vi "FipsAdjacent.vi"() -> (11 "Fips":i32[](array[numeric]))   [LabVIEW 2017] (continued)
26157\n\"Schoolcraft County, MI\"\t26153\t\"Alger County, MI\"\t26003\n\"Schoolcraft County, MI\"\t26153\t\"Charlevoix County, MI\"\t26029\n\"Schoolcraft County, MI\"\t26153\t\"Delta County, MI\"\t26041\n\"Schoolcraft County, MI\"\t26153\t\"Leelanau County, MI\"\t26089\n\"Schoolcraft County, MI\"\t26153\t\"Luce County, MI\"\t26095\n\"Schoolcraft County, MI\"\t26153\t\"Mackinac County, MI\"\t26097\n\"Schoolcraft County, MI\"\t26153\t\"Schoolcraft County, MI\"\t26153\n\"Shiawassee County, MI\"\t26155\t\"Clinton County, MI\"\t26037\n\"Shiawassee County, MI\"\t26155\t\"Genesee County, MI\"\t26049\n\"Shiawassee County, MI\"\t26155\t\"Gratiot County, MI\"\t26057\n\"Shiawassee County, MI\"\t26155\t\"Ingham County, MI\"\t26065\n\"Shiawassee County, MI\"\t26155\t\"Livingston County, MI\"\t26093\n\"Shiawassee County, MI\"\t26155\t\"Saginaw County, MI\"\t26145\n\"Shiawassee County, MI\"\t26155\t\"Shiawassee County, MI\"\t26155\n\"Tuscola County, MI\"\t26157\t\"Bay County, MI\"\t26017\n\"Tuscola County, MI\"\t26157\t\"Genesee County, MI\"\t26049\n\"Tuscola County, MI\"\t26157\t\"Huron County, MI\"\t26063\n\"Tuscola County, MI\"\t26157\t\"Lapeer County, MI\"\t26087\n\"Tuscola County, MI\"\t26157\t\"Saginaw County, MI\"\t26145\n\"Tuscola County, MI\"\t26157\t\"Sanilac County, MI\"\t26151\n\"Tuscola County, MI\"\t26157\t\"Tuscola County, MI\"\t26157\n\"Van Buren County, MI\"\t26159\t\"Lake County, IL\"\t17097\n\"Van Buren County, MI\"\t26159\t\"Allegan County, MI\"\t26005\n\"Van Buren County, MI\"\t26159\t\"Berrien County, MI\"\t26021\n\"Van Buren County, MI\"\t26159\t\"Cass County, MI\"\t26027\n\"Van Buren County, MI\"\t26159\t\"Kalamazoo County, MI\"\t26077\n\"Van Buren County, MI\"\t26159\t\"St. Joseph County, MI\"\t26149\n\"Van Buren County, MI\"\t26159\t\"Van Buren County, MI\"\t26159\n\"Washtenaw County, MI\"\t26161\t\"Jackson County, MI\"\t26075\n\"Washtenaw County, MI\"\t26161\t\"Lenawee County, MI\"\t26091\n\"Washtenaw County, MI\"\t26161\t\"Livingston County, MI\"\t26093\n\"Washtenaw County, MI\"\t26161\t\"Monroe County, MI\"\t26115\n\"Washtenaw County, MI\"\t26161\t\"Oakland County, MI\"\t26125\n\"Washtenaw County, MI\"\t26161\t\"Washtenaw County, MI\"\t26161\n\"Washtenaw County, MI\"\t26161\t\"Wayne County, MI\"\t26163\n\"Wayne County, MI\"\t26163\t\"Macomb County, MI\"\t26099\n\"Wayne County, MI\"\t26163\t\"Monroe County, MI\"\t26115\n\"Wayne County, MI\"\t26163\t\"Oakland County, MI\"\t26125\n\"Wayne County, MI\"\t26163\t\"Washtenaw County, MI\"\t26161\n\"Wayne County, MI\"\t26163\t\"Wayne County, MI\"\t26163\n\"Wexford County, MI\"\t26165\t\"Benzie County, MI\"\t26019\n\"Wexford County, MI\"\t26165\t\"Grand Traverse County, MI\"\t26055\n\"Wexford County, MI\"\t26165\t\"Kalkaska County, MI\"\t26079\n\"Wexford County, MI\"\t26165\t\"Lake County, MI\"\t26085\n\"Wexford County, MI\"\t26165\t\"Manistee County, MI\"\t26101\n\"Wexford County, MI\"\t26165\t\"Missaukee County, MI\"\t26113\n\"Wexford County, MI\"\t26165\t\"Osceola County, MI\"\t26133\n\"Wexford County, MI\"\t26165\t\"Wexford County, MI\"\t26165\n\"Aitkin County, MN\"\t27001\t\"Aitkin County, MN\"\t27001\n\"Aitkin County, MN\"\t27001\t\"Carlton County, MN\"\t27017\n\"Aitkin County, MN\"\t27001\t\"Cass County, MN\"\t27021\n\"Aitkin County, MN\"\t27001\t\"Crow Wing County, MN\"\t27035\n\"Aitkin County, MN\"\t27001\t\"Itasca County, MN\"\t27061\n\"Aitkin County, MN\"\t27001\t\"Kanabec County, MN\"\t27065\n\"Aitkin County, MN\"\t27001\t\"Mille Lacs County, MN\"\t27095\n\"Aitkin County, MN\"\t27001\t\"Pine County, MN\"\t27115\n\"Aitkin County, MN\"\t27001\t\"St. Louis County, MN\"\t27137\n\"Anoka County, MN\"\t27003\t\"Anoka County, MN\"\t27003\n\"Anoka County, MN\"\t27003\t\"Chisago County, MN\"\t27025\n\"Anoka County, MN\"\t27003\t\"Hennepin County, MN\"\t27053\n\"Anoka County, MN\"\t27003\t\"Isanti County, MN\"\t27059\n\"Anoka County, MN\"\t27003\t\"Ramsey County, MN\"\t27123\n\"Anoka County, MN\"\t27003\t\"Sherburne County, MN\"\t27141\n\"Anoka County, MN\"\t27003\t\"Washington County, MN\"\t27163\n\"Becker County, MN\"\t27005\t\"Becker County, MN\"\t27005\n\"Becker County, MN\"\t27005\t\"Clay County, MN\"\t27027\n\"Becker County, MN\"\t27005\t\"Clearwater County, MN\"\t27029\n\"Becker County, MN\"\t27005\t\"Hubbard County, MN\"\t27057\n\"Becker County, MN\"\t27005\t\"Mahnomen County, MN\"\t27087\n\"Becker County, MN\"\t27005\t\"Norman County, MN\"\t27107\n\"Becker County, MN\"\t27005\t\"Otter Tail County, MN\"\t27111\n\"Becker County, MN\"\t27005\t\"Wadena County, MN\"\t27159\n\"Beltrami County, MN\"\t27007\t\"Beltrami County, MN\"\t27007\n\"Beltrami County, MN\"\t27007\t\"Cass County, MN\"\t27021\n\"Beltrami County, MN\"\t27007\t\"Clearwater County, MN\"\t27029\n\"Beltrami County, MN\"\t27007\t\"Hubbard County, MN\"\t27057\n\"Beltrami County, MN\"\t27007\t\"Itasca County, MN\"\t27061\n\"Beltrami County, MN\"\t27007\t\"Koochiching County, MN\"\t27071\n\"Beltrami County, MN\"\t27007\t\"Lake of the Woods County, MN\"\t27077\n\"Beltrami County, MN\"\t27007\t\"Marshall County, MN\"\t27089\n\"Beltrami County, MN\"\t27007\t\"Pennington County, MN\"\t27113\n\"Beltrami County, MN\"\t27007\t\"Roseau County, MN\"\t27135\n\"Benton County, MN\"\t27009\t\"Benton County, MN\"\t27009\n\"Benton County, MN\"\t27009\t\"Mille Lacs County, MN\"\t27095\n\"Benton County, MN\"\t27009\t\"Morrison County, MN\"\t27097\n\"Benton County, MN\"\t27009\t\"Sherburne County, MN\"\t27141\n\"Benton County, MN\"\t27009\t\"Stearns County, MN\"\t27145\n\"Big Stone County, MN\"\t27011\t\"Big Stone County, MN\"\t27011\n\"Big Stone County, MN\"\t27011\t\"Lac qui Parle County, MN\"\t27073\n\"Big Stone County, MN\"\t27011\t\"Stevens County, MN\"\t27149\n\"Big Stone County, MN\"\t27011\t\"Swift County, MN\"\t27151\n\"Big Stone County, MN\"\t27011\t\"Traverse County, MN\"\t27155\n\"Big Stone County, MN\"\t27011\t\"Grant County, SD\"\t46051\n\"Big Stone County, MN\"\t27011\t\"Roberts County, SD\"\t46109\n\"Blue Earth County, MN\"\t27013\t\"Blue Earth County, MN\"\t27013\n\"Blue Earth County, MN\"\t27013\t\"Brown County, MN\"\t27015\n\"Blue Earth County, MN\"\t27013\t\"Faribault County, MN\"\t27043\n\"Blue Earth County, MN\"\t27013\t\"Le Sueur County, MN\"\t27079\n\"Blue Earth County, MN\"\t27013\t\"Martin County, MN\"\t27091\n\"Blue Earth County, MN\"\t27013\t\"Nicollet County, MN\"\t27103\n\"Blue Earth County, MN\"\t27013\t\"Waseca County, MN\"\t27161\n\"Blue Earth County, MN\"\t27013\t\"Watonwan County, MN\"\t27165\n\"Brown County, MN\"\t27015\t\"Blue Earth County, MN\"\t27013\n\"Brown County, MN\"\t27015\t\"Brown County, MN\"\t27015\n\"Brown County, MN\"\t27015\t\"Cottonwood County, MN\"\t27033\n\"Brown County, MN\"\t27015\t\"Nicollet County, MN\"\t27103\n\"Brown County, MN\"\t27015\t\"Redwood County, MN\"\t27127\n\"Brown County, MN\"\t27015\t\"Renville County, MN\"\t27129\n\"Brown County, MN\"\t27015\t\"Watonwan County, MN\"\t27165\n\"Carlton County, MN\"\t27017\t\"Aitkin County, MN\"\t27001\n\"Carlton County, MN\"\t27017\t\"Carlton County, MN\"\t27017\n\"Carlton County, MN\"\t27017\t\"Pine County, MN\"\t27115\n\"Carlton County, MN\"\t27017\t\"St. Louis County, MN\"\t27137\n\"Carlton County, MN\"\t27017\t\"Douglas County, WI\"\t55031\n\"Carver County, MN\"\t27019\t\"Carver County, MN\"\t27019\n\"Carver County, MN\"\t27019\t\"Hennepin County, MN\"\t27053\n\"Carver County, MN\"\t27019\t\"McLeod County, MN\"\t27085\n\"Carver County, MN\"\t27019\t\"Scott County, MN\"\t27139\n\"Carver County, MN\"\t27019\t\"Sibley County, MN\"\t27143\n\"Carver County, MN\"\t27019\t\"Wright County, MN\"\t27171\n\"Cass County, MN\"\t27021\t\"Aitkin County, MN\"\t27001\n\"Cass County, MN\"\t27021\t\"Beltrami County, MN\"\t27007\n\"Cass County, MN\"\t27021\t\"Cass County, MN\"\t27021\n\"Cass County, MN\"\t27021\t\"Crow Wing County, MN\"\t27035\n\"Cass County, MN\"\t27021\t\"Hubbard County, MN\"\t27057\n\"Cass County, MN\"\t27021\t\"Itasca County, MN\"\t27061\n\"Cass County, MN\"\t27021\t\"Morrison County, MN\"\t27097\n\"Cass County, MN\"\t27021\t\"Todd County, MN\"\t27153\n\"Cass County, MN\"\t27021\t\"Wadena County, MN\"\t27159\n\"Chippewa County, MN\"\t27023\t\"Chippewa County, MN\"\t27023\n\"Chippewa County, MN\"\t27023\t\"Kandiyohi County, MN\"\t27067\n\"Chippewa County, MN\"\t27023\t\"Lac qui Parle County, MN\"\t27073\n\"Chippewa County, MN\"\t27023\t\"Renville County, MN\"\t27129\n\"Chippewa County, MN\"\t27023\t\"Swift County, MN\"\t27151\n\"Chippewa County, MN\"\t27023\t\"Yellow Medicine County, MN\"\t27173\n\"Chisago County, MN\"\t27025\t\"Anoka County, MN\"\t27003\n\"Chisago County, MN\"\t27025\t\"Chisago County, MN\"\t27025\n\"Chisago County, MN\"\t27025\t\"Isanti County, MN\"\t27059\n\"Chisago County, MN\"\t27025\t\"Kanabec County, MN\"\t27065\n\"Chisago County, MN\"\t27025\t\"Pine County, MN\"\t27115\n\"Chisago County, MN\"\t27025\t\"Washington County, MN\"\t27163\n\"Chisago County, MN\"\t27025\t\"Burnett County, WI\"\t55013\n\"Chisago County, MN\"\t27025\t\"Polk County, WI\"\t55095\n\"Clay County, MN\"\t27027\t\"Becker County, MN\"\t27005\n\"Clay County, MN\"\t27027\t\"Clay County, MN\"\t27027\n\"Clay County, MN\"\t27027\t\"Norman County, MN\"\t27107\n\"Clay County, MN\"\t27027\t\"Otter Tail County, MN\"\t27111\n\"Clay County, MN\"\t27027\t\"Wilkin County, MN\"\t27167\n\"Clay County, MN\"\t27027\t\"Cass County, ND\"\t38017\n\"Clay County, MN\"\t27027\t\"Richland County, ND\"\t38077\n\"Clearwater County, MN\"\t27029\t\"Becker County, MN\"\t27005\n\"Clearwater County, MN\"\t27029\t\"Beltrami County, MN\"\t27007\n\"Clearwater County, MN\"\t27029\t\"Clearwater County, MN\"\t27029\n\"Clearwater County, MN\"\t27029\t\"Hubbard County, MN\"\t27057\n\"Clearwater County, MN\"\t27029\t\"Mahnomen County, MN\"\t27087\n\"Clearwater County, MN\"\t27029\t\"Pennington County, MN\"\t27113\n\"Clearwater County, MN\"\t27029\t\"Polk County, MN\"\t27119\n\"Cook County, MN\"\t27031\t\"Keweenaw County, MI\"\t26083\n\"Cook County, MN\"\t27031\t\"Ontonagon County, MI\"\t26131\n\"Cook County, MN\"\t27031\t\"Cook County, MN\"\t27031\n\"Cook County, MN\"\t27031\t\"Lake County, MN\"\t27075\n\"Cook County, MN\"\t27031\t\"Ashland County, WI\"\t55003\n\"Cottonwood County, MN\"\t27033\t\"Brown County, MN\"\t27015\n\"Cottonwood County, MN\"\t27033\t\"Cottonwood County, MN\"\t27033\n\"Cottonwood County, MN\"\t27033\t\"Jackson County, MN\"\t27063\n\"Cottonwood County, MN\"\t27033\t\"Murray County, MN\"\t27101\n\"Cottonwood County, MN\"\t27033\t\"Nobles County, MN\"\t27105\n\"Cottonwood County, MN\"\t27033\t\"Redwood County, MN\"\t27127\n\"Cottonwood County, MN\"\t27033\t\"Watonwan County, MN\"\t27165\n\"Crow Wing County, MN\"\t27035\t\"Aitkin County, MN\"\t27001\n\"Crow Wing County, MN\"\t27035\t\"Cass County, MN\"\t27021\n\"Crow Wing County, MN\"\t27035\t\"Crow Wing County, MN\"\t27035\n\"Crow Wing County, MN\"\t27035\t\"Mille Lacs County, MN\"\t27095\n\"Crow Wing County, MN\"\t27035\t\"Morrison County, MN\"\t27097\n\"Dakota County, MN\"\t27037\t\"Dakota County, MN\"\t27037\n\"Dakota County, MN\"\t27037\t\"Goodhue County, MN\"\t27049\n\"Dakota County, MN\"\t27037\t\"Hennepin County, MN\"\t27053\n\"Dakota County, MN\"\t27037\t\"Ramsey County, MN\"\t27123\n\"Dakota County, MN\"\t27037\t\"Rice County, MN\"\t27131\n\"Dakota County, MN\"\t27037\t\"Scott County, MN\"\t27139\n\"Dakota County, MN\"\t27037\t\"Washington County, MN\"\t27163\n\"Dakota County, MN\"\t27037\t\"Pierce County, WI\"\t55093\n\"Dodge County, MN\"\t27039\t\"Dodge County, MN\"\t27039\n\"Dodge County, MN\"\t27039\t\"Goodhue County, MN\"\t27049\n\"Dodge County, MN\"\t27039\t\"Mower County, MN\"\t27099\n\"Dodge County, MN\"\t27039\t\"Olmsted County, MN\"\t27109\n\"Dodge County, MN\"\t27039\t\"Rice County, MN\"\t27131\n\"Dodge County, MN\"\t27039\t\"Steele County, MN\"\t27147\n\"Douglas County, MN\"\t27041\t\"Douglas County, MN\"\t27041\n\"Douglas County, MN\"\t27041\t\"Grant County, MN\"\t27051\n\"Douglas County, MN\"\t27041\t\"Otter Tail County, MN\"\t27111\n\"Douglas County, MN\"\t27041\t\"Pope County, MN\"\t27121\n\"Douglas County, MN\"\t27041\t\"Stearns County, MN\"\t27145\n\"Douglas County, MN\"\t27041\t\"Stevens County, MN\"\t27149\n\"Douglas County, MN\"\t27041\t\"Todd County, MN\"\t27153\n\"Faribault County, MN\"\t27043\t\"Kossuth County, IA\"\t19109\n\"Faribault County, MN\"\t27043\t\"Winnebago County, IA\"\t19189\n\"Faribault County, MN\"\t27043\t\"Blue Earth County, MN\"\t27013\n\"Faribault County, MN\"\t27043\t\"Faribault County, MN\"\t27043\n\"Faribault County, MN\"\t27043\t\"Freeborn County, MN\"\t27047\n\"Faribault County, MN\"\t27043\t\"Martin County, MN\"\t27091\n\"Faribault County, MN\"\t27043\t\"Waseca County, MN\"\t27161\n\"Fillmore County, MN\"\t27045\t\"Howard County, IA\"\t19089\n\"Fillmore County, MN\"\t27045\t\"Winneshiek County, IA\"\t19191\n\"Fillmore County, MN\"\t27045\t\"Fillmore County, MN\"\t27045\n\"Fillmore County, MN\"\t27045\t\"Houston County, MN\"\t27055\n\"Fillmore County, MN\"\t27045\t\"Mower County, MN\"\t27099\n\"Fillmore County, MN\"\t27045\t\"Olmsted County, MN\"\t27109\n\"Fillmore County, MN\"\t27045\t\"Winona County, MN\"\t27169\n\"Freeborn County, MN\"\t27047\t\"Winnebago County, IA\"\t19189\n\"Freeborn County, MN\"\t27047\t\"Worth County, IA\"\t19195\n\"Freeborn County, MN\"\t27047\t\"Faribault County, MN\"\t27043\n\"Freeborn County, MN\"\t27047\t\"Freeborn County, MN\"\t27047\n\"Freeborn County, MN\"\t27047\t\"Mower County, MN\"\t27099\n\"Freeborn County, MN\"\t27047\t\"Steele County, MN\"\t27147\n\"Freeborn County, MN\"\t27047\t\"Waseca County, MN\"\t27161\n\"Goodhue County, MN\"\t27049\t\"Dakota County, MN\"\t27037\n\"Goodhue County, MN\"\t27049\t\"Dodge County, MN\"\t27039\n\"Goodhue County, MN\"\t27049\t\"Goodhue County, MN\"\t27049\n\"Goodhue County, MN\"\t27049\t\"Olmsted County, MN\"\t27109\n\"Goodhue County, MN\"\t27049\t\"Rice County, MN\"\t27131\n\"Goodhue County, MN\"\t27049\t\"Wabasha County, MN\"\t27157\n\"Goodhue County, MN\"\t27049\t\"Pepin County, WI\"\t55091\n\"Goodhue County, MN\"\t27049\t\"Pierce County, WI\"\t55093\n\"Grant County, MN\"\t27051\t\"Douglas County, MN\"\t27041\n\"Grant County, MN\"\t27051\t\"Grant County, MN\"\t27051\n\"Grant County, MN\"\t27051\t\"Otter Tail County, MN\"\t27111\n\"Grant County, MN\"\t27051\t\"Pope County, MN\"\t27121\n\"Grant County, MN\"\t27051\t\"Stevens County, MN\"\t27149\n\"Grant County, MN\"\t27051\t\"Traverse County, MN\"\t27155\n\"Grant County, MN\"\t27051\t\"Wilkin County, MN\"\t27167\n\"Hennepin County, MN\"\t27053\t\"Anoka County, MN\"\t27003\n\"Hennepin County, MN\"\t27053\t\"Carver County, MN\"\t27019\n\"Hennepin County, MN\"\t27053\t\"Dakota County, MN\"\t27037\n\"Hennepin County, MN\"\t27053\t\"Hennepin County, MN\"\t27053\n\"Hennepin County, MN\"\t27053\t\"Ramsey County, MN\"\t27123\n\"Hennepin County, MN\"\t27053\t\"Scott County, MN\"\t27139\n\"Hennepin County, MN\"\t27053\t\"Sherburne County, MN\"\t27141\n\"Hennepin County, MN\"\t27053\t\"Wright County, MN\"\t27171\n\"Houston County, MN\"\t27055\t\"Allamakee County, IA\"\t19005\n\"Houston County, MN\"\t27055\t\"Winneshiek County, IA\"\t19191\n\"Houston County, MN\"\t27055\t\"Fillmore County, MN\"\t27045\n\"Houston County, MN\"\t27055\t\"Houston County, MN\"\t27055\n\"Houston County, MN\"\t27055\t\"Winona County, MN\"\t27169\n\"Houston County, MN\"\t27055\t\"La Crosse County, WI\"\t55063\n\"Houston County, MN\"\t27055\t\"Vernon County, WI\"\t55123\n\"Hubbard County, MN\"\t27057\t\"Becker County, MN\"\t27005\n\"Hubbard County, MN\"\t27057\t\"Beltrami County, MN\"\t27007\n\"Hubbard County, MN\"\t27057\t\"Cass County, MN\"\t27021\n\"Hubbard County, MN\"\t27057\t\"Clearwater County, MN\"\t27029\n\"Hubbard County, MN\"\t27057\t\"Hubbard County, MN\"\t27057\n\"Hubbard County, MN\"\t27057\t\"Wadena County, MN\"\t27159\n\"Isanti County, MN\"\t27059\t\"Anoka County, MN\"\t27003\n\"Isanti County, MN\"\t27059\t\"Chisago County, MN\"\t27025\n\"Isanti County, MN\"\t27059\t\"Isanti County, MN\"\t27059\n\"Isanti County, MN\"\t27059\t\"Kanabec County, MN\"\t27065\n\"Isanti County, MN\"\t27059\t\"Mille Lacs County, MN\"\t27095\n\"Isanti County, MN\"\t27059\t\"Pine County, MN\"\t27115\n\"Isanti County, MN\"\t27059\t\"Sherburne County, MN\"\t27141\n\"Itasca County, MN\"\t27061\t\"Aitkin County, MN\"\t27001\n\"Itasca County, MN\"\t27061\t\"Beltrami County, MN\"\t27007\n\"Itasca County, MN\"\t27061\t\"Cass County, MN\"\t27021\n\"Itasca County, MN\"\t27061\t\"Itasca County, MN\"\t27061\n\"Itasca County, MN\"\t27061\t\"Koochiching County, MN\"\t27071\n\"Itasca County, MN\"\t27061\t\"St. Louis County, MN\"\t27137\n\"Jackson County, MN\"\t27063\t\"Dickinson County, IA\"\t19059\n\"Jackson County, MN\"\t27063\t\"Emmet County, IA\"\t19063\n\"Jackson County, MN\"\t27063\t\"Osceola County, IA\"\t19143\n\"Jackson County, MN\"\t27063\t\"Cottonwood County, MN\"\t27033\n\"Jackson County, MN\"\t27063\t\"Jackson County, MN\"\t27063\n\"Jackson County, MN\"\t27063\t\"Martin County, MN\"\t27091\n\"Jackson County, MN\"\t27063\t\"Nobles County, MN\"\t27105\n\"Jackson County, MN\"\t27063\t\"Watonwan County, MN\"\t27165\n\"Kanabec County, MN\"\t27065\t\"Aitkin County, MN\"\t27001\n\"Kanabec County, MN\"\t27065\t\"Chisago County, MN\"\t27025\n\"Kanabec County, MN\"\t27065\t\"Isanti County, MN\"\t27059\n\"Kanabec County, MN\"\t27065\t\"Kanabec County, MN\"\t27065\n\"Kanabec County, MN\"\t27065\t\"Mille Lacs County, MN\"\t27095\n\"Kanabec County, MN\"\t27065\t\"Pine County, MN\"\t27115\n\"Kandiyohi County, MN\"\t27067\t\"Chippewa County, MN\"\t27023\n\"Kandiyohi County, MN\"\t27067\t\"Kandiyohi County, MN\"\t27067\n\"Kandiyohi County, MN\"\t27067\t\"Meeker County, MN\"\t27093\n\"Kandiyohi County, MN\"\t27067\t\"Pope County, MN\"\t27121\n\"Kandiyohi County, MN\"\t27067\t\"Renville County, MN\"\t27129\n\"Kandiyohi County, MN\"\t27067\t\"Stearns County, MN\"\t27145\n\"Kandiyohi County, MN\"\t27067\t\"Swift County, MN\"\t27151\n\"Kittson County, MN\"\t27069\t\"Kittson County, MN\"\t27069\n\"Kittson County, MN\"\t27069\t\"Marshall County, MN\"\t27089\n\"Kittson County, MN\"\t27069\t\"Roseau County, MN\"\t27135\n\"Kittson County, MN\"\t27069\t\"Pembina County, ND\"\t38067\n\"Koochiching County, MN\"\t27071\t\"Beltrami County, MN\"\t27007\n\"Koochiching County, MN\"\t27071\t\"Itasca County, MN\"\t27061\n\"Koochiching County, MN\"\t27071\t\"Koochiching County, MN\"\t27071\n\"Koochiching County, MN\"\t27071\t\"Lake of the Woods County, MN\"\t27077\n\"Koochiching County, MN\"\t27071\t\"St. Louis County, MN\"\t27137\n\"Lac qui Parle County, MN\"\t27073\t\"Big Stone County, MN\"\t27011\n\"Lac qui Parle County, MN\"\t27073\t\"Chippewa County, MN\"\t27023\n\"Lac qui Parle County, MN\"\t27073\t\"Lac qui Parle County, MN\"\t27073\n\"Lac qui Parle County, MN\"\t27073\t\"Swift County, MN\"\t27151\n\"Lac qui Parle County, MN\"\t27073\t\"Yellow Medicine County, MN\"\t27173\n\"Lac qui Parle County, MN\"\t27073\t\"Deuel County, SD\"\t46039\n\"Lac qui Parle County, MN\"\t27073\t\"Grant County, SD\"\t46051\n\"Lake County, MN\"\t27075\t\"Cook County, MN\"\t27031\n\"Lake County, MN\"\t27075\t\"Lake County, MN\"\t27075\n\"Lake County, MN\"\t27075\t\"St. Louis County, MN\"\t27137\n\"Lake County, MN\"\t27075\t\"Ashland County, WI\"\t55003\n\"Lake County, MN\"\t27075\t\"Bayfield County, WI\"\t55007\n\"Lake County, MN\"\t27075\t\"Douglas County, WI\"\t55031\n\"Lake of the Woods County, MN\"\t27077\t\"Beltrami County, MN\"\t27007\n\"Lake of the Woods County, MN\"\t27077\t\"Koochiching County, MN\"\t27071\n\"Lake of the Woods County, MN\"\t27077\t\"Lake of the Woods County, MN\"\t27077\n\"Lake of the Woods County, MN\"\t27077\t\"Roseau County, MN\"\t27135\n\"Le Sueur County, MN\"\t27079\t\"Blue Earth County, MN\"\t27013\n\"Le Sueur County, MN\"\t27079\t\"Le Sueur County, MN\"\t27079\n\"Le Sueur County, MN\"\t27079\t\"Nicollet County, MN\"\t27103\n\"Le Sueur County, MN\"\t27079\t\"Rice County, MN\"\t27131\n\"Le Sueur County, MN\"\t27079\t\"Scott County, MN\"\t27139\n\"Le Sueur County, MN\"\t27079\t\"Sibley County, MN\"\t27143\n\"Le Sueur County, MN\"\t27079\t\"Waseca County, MN\"\t27161\n\"Lincoln County, MN\"\t27081\t\"Lincoln County, MN\"\t27081\n\"Lincoln County, MN\"\t27081\t\"Lyon County, MN\"\t27083\n\"Lincoln County, MN\"\t27081\t\"Pipestone County, MN\"\t27117\n\"Lincoln County, MN\"\t27081\t\"Yellow Medicine County, MN\"\t27173\n\"Lincoln County, MN\"\t27081\t\"Brookings County, SD\"\t46011\n\"Lincoln County, MN\"\t27081\t\"Deuel County, SD\"\t46039\n\"Lincoln County, MN\"\t27081\t\"Moody County, SD\"\t46101\n\"Lyon County, MN\"\t27083\t\"Lincoln County, MN\"\t27081\n\"Lyon County, MN\"\t27083\t\"Lyon County, MN\"\t27083\n\"Lyon County, MN\"\t27083\t\"Murray County, MN\"\t27101\n\"Lyon County, MN\"\t27083\t\"Pipestone County, MN\"\t27117\n\"Lyon County, MN\"\t27083\t\"Redwood County, MN\"\t27127\n\"Lyon County, MN\"\t27083\t\"Yellow Medicine County, MN\"\t27173\n\"McLeod County, MN\"\t27085\t\"Carver County, MN\"\t27019\n\"McLeod County, MN\"\t27085\t\"McLeod County, MN\"\t27085\n\"McLeod County, MN\"\t27085\t\"Meeker County, MN\"\t27093\n\"McLeod County, MN\"\t27085\t\"Renville County, MN\"\t27129\n\"McLeod County, MN\"\t27085\t\"Sibley County, MN\"\t27143\n\"McLeod County, MN\"\t27085\t\"Wright County, MN\"\t27171\n\"Mahnomen County, MN\"\t27087\t\"Becker County, MN\"\t27005\n\"Mahnomen County, MN\"\t27087\t\"Clearwater County, MN\"\t27029\n\"Mahnomen County, MN\"\t27087\t\"Mahnomen County, MN\"\t27087\n\"Mahnomen County, MN\"\t27087\t\"Norman County, MN\"\t27107\n\"Mahnomen County, MN\"\t27087\t\"Polk County, MN\"\t27119\n\"Marshall County, MN\"\t27089\t\"Beltrami County, MN\"\t27007\n\"Marshall County, MN\"\t27089\t\"Kittson County, MN\"\t27069\n\"Marshall County, MN\"\t27089\t\"Marshall County, MN\"\t27089\n\"Marshall County, MN\"\t27089\t\"Pennington County, MN\"\t27113\n\"Marshall County, MN\"\t27089\t\"Polk County, MN\"\t27119\n\"Marshall County, MN\"\t27089\t\"Roseau County, MN\"\t27135\n\"Marshall County, MN\"\t27089\t\"Grand Forks County, ND\"\t38035\n\"Marshall County, MN\"\t27089\t\"Pembina County, ND\"\t38067\n\"Marshall County, MN\"\t27089\t\"Walsh County, ND\"\t38099\n\"Martin County, MN\"\t27091\t\"Emmet County, IA\"\t19063\n\"Martin County, MN\"\t27091\t\"Kossuth County, IA\"\t19109\n\"Martin County, MN\"\t27091\t\"Blue Earth County, MN\"\t27013\n\"Martin County, MN\"\t27091\t\"Faribault County, MN\"\t27043\n\"Martin County, MN\"\t27091\t\"Jackson County, MN\"\t27063\n\"Martin County, MN\"\t27091\t\"Martin County, MN\"\t27091\n\"Martin County, MN\"\t27091\t\"Watonwan County, MN\"\t27165\n\"Meeker County, MN\"\t27093\t\"Kandiyohi County, MN\"\t27067\n\"Meeker County, MN\"\t27093\t\"McLeod County, MN\"\t27085\n\"Meeker County, MN\"\t27093\t\"Meeker County, MN\"\t27093\n\"Meeker County, MN\"\t27093\t\"Renville County, MN\"\t27129\n\"Meeker County, MN\"\t27093\t\"Stearns County, MN\"\t27145\n\"Meeker County, MN\"\t27093\t\"Wright County, MN\"\t27171\n\"Mille Lacs County, MN\"\t27095\t\"Aitkin County, MN\"\t27001\n\"Mille Lacs County, MN\"\t27095\t\"Benton County, MN\"\t27009\n\"Mille Lacs County, MN\"\t27095\t\"Crow Wing County, MN\"\t27035\n\"Mille Lacs County, MN\"\t27095\t\"Isanti County, MN\"\t27059\n\"Mille Lacs County, MN\"\t27095\t\"Kanabec County, MN\"\t27065\n\"Mille Lacs County, MN\"\t27095\t\"Mille Lacs County, MN\"\t27095\n\"Mille Lacs County, MN\"\t27095\t\"Morrison County, MN\"\t27097\n\"Mille Lacs County, MN\"\t27095\t\"Sherburne County, MN\"\t27141\n\"Morrison County, MN\"\t27097\t\"Benton County, MN\"\t27009\n\"Morrison County, MN\"\t27097\t\"Cass County, MN\"\t27021\n\"Morrison County, MN\"\t27097\t\"Crow Wing County, MN\"\t27035\n\"Morrison County, MN\"\t27097\t\"Mille Lacs County, MN\"\t27095\n\"Morrison County, MN\"\t27097\t\"Morrison County, MN\"\t27097\n\"Morrison County, MN\"\t27097\t\"Stearns County, MN\"\t27145\n\"Morrison County, MN\"\t27097\t\"Todd County, MN\"\t27153\n\"Mower County, MN\"\t27099\t\"Howard County, IA\"\t19089\n\"Mower County, MN\"\t27099\t\"Mitchell County, IA\"\t19131\n\"Mower County, MN\"\t27099\t\"Worth County, IA\"\t19195\n\"Mower County, MN\"\t27099\t\"Dodge County, MN\"\t27039\n\"Mower County, MN\"\t27099\t\"Fillmore County, MN\"\t27045\n\"Mower County, MN\"\t27099\t\"Freeborn County, MN\"\t27047\n\"Mower County, MN\"\t27099\t\"Mower County, MN\"\t27099\n\"Mower County, MN\"\t27099\t\"Olmsted County, MN\"\t27109\n\"Mower County, MN\"\t27099\t\"Steele County, MN\"\t27147\n\"Murray County, MN\"\t27101\t\"Cottonwood County, MN\"\t27033\n\"Murray County, MN\"\t27101\t\"Lyon County, MN\"\t27083\n\"Murray County, MN\"\t27101\t\"Murray County, MN\"\t27101\n\"Murray County, MN\"\t27101\t\"Nobles County, MN\"\t27105\n\"Murray County, MN\"\t27101\t\"Pipestone County, MN\"\t27117\n\"Murray County, MN\"\t27101\t\"Redwood County, MN\"\t27127\n\"Murray County, MN\"\t27101\t\"Rock County, MN\"\t27133\n\"Nicollet County, MN\"\t27103\t\"Blue Earth County, MN\"\t27013\n\"Nicollet County, MN\"\t27103\t\"Brown County, MN\"\t27015\n\"Nicollet County, MN\"\t27103\t\"Le Sueur County, MN\"\t27079\n\"Nicollet County, MN\"\t27103\t\"Nicollet County, MN\"\t27103\n\"Nicollet County, MN\"\t27103\t\"Renville County, MN\"\t27129\n\"Nicollet County, MN\"\t27103\t\"Sibley County, MN\"\t27143\n\"Nobles County, MN\"\t27105\t\"Lyon County, IA\"\t19119\n\"Nobles County, MN\"\t27105\t\"Osceola County, IA\"\t19143\n\"Nobles County, MN\"\t27105\t\"Cottonwood County, MN\"\t27033\n\"Nobles County, MN\"\t27105\t\"Jackson County, MN\"\t27063\n\"Nobles County, MN\"\t27105\t\"Murray County, MN\"\t27101\n\"Nobles County, MN\"\t27105\t\"Nobles County, MN\"\t27105\n\"Nobles County, MN\"\t27105\t\"Rock County, MN\"\t27133\n\"Norman County, MN\"\t27107\t\"Becker County, MN\"\t27005\n\"Norman County, MN\"\t27107\t\"Clay County, MN\"\t27027\n\"Norman County, MN\"\t27107\t\"Mahnomen County, MN\"\t27087\n\"Norman County, MN\"\t27107\t\"Norman County, MN\"\t27107\n\"Norman County, MN\"\t27107\t\"Polk County, MN\"\t27119\n\"Norman County, MN\"\t27107\t\"Cass County, ND\"\t38017\n\"Norman County, MN\"\t27107\t\"Traill County, ND\"\t38097\n\"Olmsted County, MN\"\t27109\t\"Dodge County, MN\"\t27039\n\"Olmsted County, MN\"\t27109\t\"Fillmore County, MN\"\t27045\n\"Olmsted County, MN\"\t27109\t\"Goodhue County, MN\"\t27049\n\"Olmsted County, MN\"\t27109\t\"Mower County, MN\"\t27099\n\"Olmsted County, MN\"\t27109\t\"Olmsted County, MN\"\t27109\n\"Olmsted County, MN\"\t27109\t\"Wabasha County, MN\"\t27157\n\"Olmsted County, MN\"\t27109\t\"Winona County, MN\"\t27169\n\"Todd County, MN\"\t27111\t\"Becker County, MN\"\t27005\n\"Todd County, MN\"\t27111\t\"Clay County, MN\"\t27027\n\"Todd County, MN\"\t27111\t\"Douglas County, MN\"\t27041\n\"Todd County, MN\"\t27111\t\"Grant County, MN\"\t27051\n\"Todd County, MN\"\t27111\t\"Otter Tail County, MN\"\t27111\n\"Todd County, MN\"\t27111\t\"Todd County, MN\"\t27153\n\"Todd County, MN\"\t27111\t\"Wadena County, MN\"\t27159\n\"Todd County, MN\"\t27111\t\"Wilkin County, MN\"\t27167\n\"Pennington County, MN\"\t27113\t\"Beltrami County, MN\"\t27007\n\"Pennington County, MN\"\t27113\t\"Clearwater County, MN\"\t27029\n\"Pennington County, MN\"\t27113\t\"Marshall County, MN\"\t27089\n\"Pennington County, MN\"\t27113\t\"Pennington County, MN\"\t27113\n\"Pennington County, MN\"\t27113\t\"Polk County, MN\"\t27119\n\"Pennington County, MN\"\t27113\t\"Red Lake County, MN\"\t27125\n\"Pine County, MN\"\t27115\t\"Aitkin County, MN\"\t27001\n\"Pine County, MN\"\t27115\t\"Carlton County, MN\"\t27017\n\"Pine County, MN\"\t27115\t\"Chisago County, MN\"\t27025\n\"Pine County, MN\"\t27115\t\"Isanti County, MN\"\t27059\n\"Pine County, MN\"\t27115\t\"Kanabec County, MN\"\t27065\n\"Pine County, MN\"\t27115\t\"Pine County, MN\"\t27115\n\"Pine County, MN\"\t27115\t\"Burnett County, WI\"\t55013\n\"Pine County, MN\"\t27115\t\"Douglas County, WI\"\t55031\n\"Pipestone County, MN\"\t27117\t\"Lincoln County, MN\"\t27081\n\"Pipestone County, MN\"\t27117\t\"Lyon County, MN\"\t27083\n\"Pipestone County, MN\"\t27117\t\"Murray County, MN\"\t27101\n\"Pipestone County, MN\"\t27117\t\"Pipestone County, MN\"\t27117\n\"Pipestone County, MN\"\t27117\t\"Rock County, MN\"\t27133\n\"Pipestone County, MN\"\t27117\t\"Brookings County, SD\"\t46011\n\"Pipestone County, MN\"\t27117\t\"Minnehaha County, SD\"\t46099\n\"Pipestone County, MN\"\t27117\t\"Moody County, SD\"\t46101\n\"Polk County, MN\"\t27119\t\"Clearwater County, MN\"\t27029\n\"Polk County, MN\"\t27119\t\"Mahnomen County, MN\"\t27087\n\"Polk County, MN\"\t27119\t\"Marshall County, MN\"\t27089\n\"Polk County, MN\"\t27119\t\"Norman County, MN\"\t27107\n\"Polk County, MN\"\t27119\t\"Pennington County, MN\"\t27113\n\"Polk County, MN\"\t27119\t\"Polk County, MN\"\t27119\n\"Polk County, MN\"\t27119\t\"Red Lake County, MN\"\t27125\n\"Polk County, MN\"\t27119\t\"Grand Forks County, ND\"\t38035\n\"Polk County, MN\"\t27119\t\"Traill County, ND\"\t38097\n\"Pope County, MN\"\t27121\t\"Douglas County, MN\"\t27041\n\"Pope County, MN\"\t27121\t\"Grant County, MN\"\t27051\n\"Pope County, MN\"\t27121\t\"Kandiyohi County, MN\"\t27067\n\"Pope County, MN\"\t27121\t\"Pope County, MN\"\t27121\n\"Pope County, MN\"\t27121\t\"Stearns County, MN\"\t27145\n\"Pope County, MN\"\t27121\t\"Stevens County, MN\"\t27149\n\"Pope County, MN\"\t27121\t\"Swift County, MN\"\t27151\n\"Ramsey County, MN\"\t27123\t\"Anoka County, MN\"\t27003\n\"Ramsey County, MN\"\t27123\t\"Dakota County, MN\"\t27037\n\"Ramsey County, MN\"\t27123\t\"Hennepin County, MN\"\t27053\n\"Ramsey County, MN\"\t27123\t\"Ramsey County, MN\"\t27123\n\"Ramsey County, MN\"\t27123\t\"Washington County, MN\"\t27163\n\"Red Lake County, MN\"\t27125\t\"Pennington County, MN\"\t27113\n\"Red Lake County, MN\"\t27125\t\"Polk County, MN\"\t27119\n\"Red Lake County, MN\"\t27125\t\"Red Lake County, MN\"\t27125\n\"Redwood County, MN\"\t27127\t\"Brown County, MN\"\t27015\n\"Redwood County, MN\"\t27127\t\"Cottonwood County, MN\"\t27033\n\"Redwood County, MN\"\t27127\t\"Lyon County, MN\"\t27083\n\"Redwood County, MN\"\t27127\t\"Murray County, MN\"\t27101\n\"Redwood County, MN\"\t27127\t\"Redwood County, MN\"\t27127\n\"Redwood County, MN\"\t27127\t\"Renville County, MN\"\t27129\n\"Redwood County, MN\"\t27127\t\"Yellow Medicine County, MN\"\t27173\n\"Renville County, MN\"\t27129\t\"Brown County, MN\"\t27015\n\"Renville County, MN\"\t27129\t\"Chippewa County, MN\"\t27023\n\"Renville County, MN\"\t27129\t\"Kandiyohi County, MN\"\t27067\n\"Renville County, MN\"\t27129\t\"McLeod County, MN\"\t27085\n\"Renville County, MN\"\t27129\t\"Meeker County, MN\"\t27093\n\"Renville County, MN\"\t27129\t\"Nicollet County, MN\"\t27103\n\"Renville County, MN\"\t27129\t\"Redwood County, MN\"\t27127\n\"Renville County, MN\"\t27129\t\"Renville County, MN\"\t27129\n\"Renville County, MN\"\t27129\t\"Sibley County, MN\"\t27143\n\"Renville County, MN\"\t27129\t\"Yellow Medicine County, MN\"\t27173\n\"Rice County, MN\"\t27131\t\"Dakota County, MN\"\t27037\n\"Rice County, MN\"\t27131\t\"Dodge County, MN\"\t27039\n\"Rice County, MN\"\t27131\t\"Goodhue County, MN\"\t27049\n\"Rice County, MN\"\t27131\t\"Le Sueur County, MN\"\t27079\n\"Rice County, MN\"\t27131\t\"Rice County, MN\"\t27131\n\"Rice County, MN\"\t27131\t\"Scott County, MN\"\t27139\n\"Rice County, MN\"\t27131\t\"Steele County, MN\"\t27147\n\"Rice County, MN\"\t27131\t\"Waseca County, MN\"\t27161\n\"Rock County, MN\"\t27133\t\"Lyon County, IA\"\t19119\n\"Rock County, MN\"\t27133\t\"Murray County, MN\"\t27101\n\"Rock County, MN\"\t27133\t\"Nobles County, MN\"\t27105\n\"Rock County, MN\"\t27133\t\"Pipestone County, MN\"\t27117\n\"Rock County, MN\"\t27133\t\"Rock County, MN\"\t27133\n\"Rock County, MN\"\t27133\t\"Minnehaha County, SD\"\t46099\n\"Rock County, MN\"\t27133\t\"Moody County, SD\"\t46101\n\"Roseau County, MN\"\t27135\t\"Beltrami County, MN\"\t27007\n\"Roseau County, MN\"\t27135\t\"Kittson County, MN\"\t27069\n\"Roseau County, MN\"\t27135\t\"Lake of the Woods County, MN\"\t27077\n\"Roseau County, MN\"\t27135\t\"Marshall County, MN\"\t27089\n\"Roseau County, MN\"\t27135\t\"Roseau County, MN\"\t27135\n\"St. Louis County, MN\"\t27137\t\"Aitkin County, MN\"\t27001\n\"St. Louis County, MN\"\t27137\t\"Carlton County, MN\"\t27017\n\"St. Louis County, MN\"\t27137\t\"Itasca County, MN\"\t27061\n\"St. Louis County, MN\"\t27137\t\"Koochiching County, MN\"\t27071\n\"St. Louis County, MN\"\t27137\t\"Lake County, MN\"\t27075\n\"St. Louis County, MN\"\t27137\t\"St. Louis County, MN\"\t27137\n\"St. Louis County, MN\"\t27137\t\"Douglas County, WI\"\t55031\n\"Scott County, MN\"\t27139\t\"Carver County, MN\"\t27019\n\"Scott County, MN\"\t27139\t\"Dakota County, MN\"\t27037\n\"Scott County, MN\"\t27139\t\"Hennepin County, MN\"\t27053\n\"Scott County, MN\"\t27139\t\"Le Sueur County, MN\"\t27079\n\"Scott County, MN\"\t27139\t\"Rice County, MN\"\t27131\n\"Scott County, MN\"\t27139\t\"Scott County, MN\"\t27139\n\"Scott County, MN\"\t27139\t\"Sibley County, MN\"\t27143\n\"Sherburne County, MN\"\t27141\t\"Anoka County, MN\"\t27003\n\"Sherburne County, MN\"\t27141\t\"Benton County, MN\"\t27009\n\"Sherburne County, MN\"\t27141\t\"Hennepin County, MN\"\t27053\n\"Sherburne County, MN\"\t27141\t\"Isanti County, MN\"\t27059\n\"Sherburne County, MN\"\t27141\t\"Mille Lacs County, MN\"\t27095\n\"Sherburne County, MN\"\t27141\t\"Sherburne County, MN\"\t27141\n\"Sherburne County, MN\"\t27141\t\"Stearns County, MN\"\t27145\n\"Sherburne County, MN\"\t27141\t\"Wright County, MN\"\t27171\n\"Sibley County, MN\"\t27143\t\"Carver County, MN\"\t27019\n\"Sibley County, MN\"\t27143\t\"Le Sueur County, MN\"\t27079\n\"Sibley County, MN\"\t27143\t\"McLeod County, MN\"\t27085\n\"Sibley County, MN\"\t27143\t\"Nicollet County, MN\"\t27103\n\"Sibley County, MN\"\t27143\t\"Renville County, MN\"\t27129\n\"Sibley County, MN\"\t27143\t\"Scott County, MN\"\t27139\n\"Sibley County, MN\"\t27143\t\"Sibley County, MN\"\t27143\n\"Stearns County, MN\"\t27145\t\"Benton County, MN\"\t27009\n\"Stearns County, MN\"\t27145\t\"Douglas County, MN\"\t27041\n\"Stearns County, MN\"\t27145\t\"Kandiyohi County, MN\"\t27067\n\"Stearns County, MN\"\t27145\t\"Meeker County, MN\"\t27093\n\"Stearns County, MN\"\t27145\t\"Morrison County, MN\"\t27097\n\"Stearns County, MN\"\t27145\t\"Pope County, MN\"\t27121\n\"Stearns County, MN\"\t27145\t\"Sherburne County, MN\"\t27141\n\"Stearns County, MN\"\t27145\t\"Stearns County, MN\"\t27145\n\"Stearns County, MN\"\t27145\t\"Todd County, MN\"\t27153\n\"Stearns County, MN\"\t27145\t\"Wright County, MN\"\t27171\n\"Steele County, MN\"\t27147\t\"Dodge County, MN\"\t27039\n\"Steele County, MN\"\t27147\t\"Freeborn County, MN\"\t27047\n\"Steele County, MN\"\t27147\t\"Mower County, MN\"\t27099\n\"Steele County, MN\"\t27147\t\"Rice County, MN\"\t27131\n\"Steele County, MN\"\t27147\t\"Steele County, MN\"\t27147\n\"Steele County, MN\"\t27147\t\"Waseca County, MN\"\t27161\n\"Stevens County, MN\"\t27149\t\"Big Stone County, MN\"\t27011\n\"Stevens County, MN\"\t27149\t\"Douglas County, MN\"\t27041\n\"Stevens County, MN\"\t27149\t\"Grant County, MN\"\t27051\n\"Stevens County, MN\"\t27149\t\"Pope County, MN\"\t27121\n\"Stevens County, MN\"\t27149\t\"Stevens County, MN\"\t27149\n\"Stevens County, MN\"\t27149\t\"Swift County, MN\"\t27151\n\"Stevens County, MN\"\t27149\t\"Traverse County, MN\"\t27155\n\"Swift County, MN\"\t27151\t\"Big Stone County, MN\"\t27011\n\"Swift County, MN\"\t27151\t\"Chippewa County, MN\"\t27023\n\"Swift County, MN\"\t27151\t\"Kandiyohi County, MN\"\t27067\n\"Swift County, MN\"\t27151\t\"Lac qui Parle County, MN\"\t27073\n\"Swift County, MN\"\t27151\t\"Pope County, MN\"\t27121\n\"Swift County, MN\"\t27151\t\"Stevens County, MN\"\t27149\n\"Swift County, MN\"\t27151\t\"Swift County, MN\"\t27151\n\"Todd County, MN\"\t27153\t\"Cass County, MN\"\t27021\n\"Todd County, MN\"\t27153\t\"Douglas County, MN\"\t27041\n\"Todd County, MN\"\t27153\t\"Morrison County, MN\"\t27097\n\"Todd County, MN\"\t27153\t\"Otter Tail County, MN\"\t27111\n\"Todd County, MN\"\t27153\t\"Stearns County, MN\"\t27145\n\"Todd County, MN\"\t27153\t\"Todd County, MN\"\t27153\n\"Todd County, MN\"\t27153\t\"Wadena County, MN\"\t27159\n\"Traverse County, MN\"\t27155\t\"Big Stone County, MN\"\t27011\n\"Traverse County, MN\"\t27155\t\"Grant County, MN\"\t27051\n\"Traverse County, MN\"\t27155\t\"Stevens County, MN\"\t27149\n\"Traverse County, MN\"\t27155\t\"Traverse County, MN\"\t27155\n\"Traverse County, MN\"\t27155\t\"Wilkin County, MN\"\t27167\n\"Traverse County, MN\"\t27155\t\"Richland County, ND\"\t38077\n\"Traverse County, MN\"\t27155\t\"Roberts County, SD\"\t46109\n\"Wabasha County, MN\"\t27157\t\"Goodhue County, MN\"\t27049\n\"Wabasha County, MN\"\t27157\t\"Olmsted County, MN\"\t27109\n\"Wabasha County, MN\"\t27157\t\"Wabasha County, MN\"\t27157\n\"Wabasha County, MN\"\t27157\t\"Winona County, MN\"\t27169\n\"Wabasha County, MN\"\t27157\t\"Buffalo County, WI\"\t55011\n\"Wabasha County, MN\"\t27157\t\"Pepin County, WI\"\t55091\n\"Wadena County, MN\"\t27159\t\"Becker County, MN\"\t27005\n\"Wadena County, MN\"\t27159\t\"Cass County, MN\"\t27021\n\"Wadena County, MN\"\t27159\t\"Hubbard County, MN\"\t27057\n\"Wadena County, MN\"\t27159\t\"Otter Tail County, MN\"\t27111\n\"Wadena County, MN\"\t27159\t\"Todd County, MN\"\t27153\n\"Wadena County, MN\"\t27159\t\"Wadena County, MN\"\t27159\n\"Waseca County, MN\"\t27161\t\"Blue Earth County, MN\"\t27013\n\"Waseca County, MN\"\t27161\t\"Faribault County, MN\"\t27043\n\"Waseca County, MN\"\t27161\t\"Freeborn County, MN\"\t27047\n\"Waseca County, MN\"\t27161\t\"Le Sueur County, MN\"\t27079\n\"Waseca County, MN\"\t27161\t\"Rice County, MN\"\t27131\n\"Waseca County, MN\"\t27161\t\"Steele County, MN\"\t27147\n\"Waseca County, MN\"\t27161\t\"Waseca County, MN\"\t27161\n\"Washington County, MN\"\t27163\t\"Anoka County, MN\"\t27003\n\"Washington County, MN\"\t27163\t\"Chisago County, MN\"\t27025\n\"Washington County, MN\"\t27163\t\"Dakota County, MN\"\t27037\n\"Washington County, MN\"\t27163\t\"Ramsey County, MN\"\t27123\n\"Washington County, MN\"\t27163\t\"Washington County, MN\"\t27163\n\"Washington County, MN\"\t27163\t\"Pierce County, WI\"\t55093\n\"Washington County, MN\"\t27163\t\"Polk County, WI\"\t55095\n\"Washington County, MN\"\t27163\t\"St. Croix County, WI\"\t55109\n\t27165\t\"Blue Earth County, MN\"\t27013\n\"Washington County, MN\"\t27163\t\"Brown County, MN\"\t27015\n\"Washington County, MN\"\t27163\t\"Cottonwood County, MN\"\t27033\n\"Washington County, MN\"\t27163\t\"Jackson County, MN\"\t27063\n\"Washington County, MN\"\t27163\t\"Martin County, MN\"\t27091\n\"Washington County, MN\"\t27163\t\"Watonwan County, MN\"\t27165\n\"Wilkin County, MN\"\t27167\t\"Clay County, MN\"\t27027\n\"Wilkin County, MN\"\t27167\t\"Grant County, MN\"\t27051\n\"Wilkin County, MN\"\t27167\t\"Otter Tail County, MN\"\t27111\n\"Wilkin County, MN\"\t27167\t\"Traverse County, MN\"\t27155\n\"Wilkin County, MN\"\t27167\t\"Wilkin County, MN\"\t27167\n\"Wilkin County, MN\"\t27167\t\"Richland County, ND\"\t38077\n\"Winona County, MN\"\t27169\t\"Fillmore County, MN\"\t27045\n\"Winona County, MN\"\t27169\t\"Houston County, MN\"\t27055\n\"Winona County, MN\"\t27169\t\"Olmsted County, MN\"\t27109\n\"Winona County, MN\"\t27169\t\"Wabasha County, MN\"\t27157\n\"Winona County, MN\"\t27169\t\"Winona County, MN\"\t27169\n\"Winona County, MN\"\t27169\t\"Buffalo County, WI\"\t55011\n\"Winona County, MN\"\t27169\t\"La Crosse County, WI\"\t55063\n\"Winona County, MN\"\t27169\t\"Trempealeau County, WI\"\t55121\n\"Wright County, MN\"\t27171\t\"Carver County, MN\"\t27019\n\"Wright County, MN\"\t27171\t\"Hennepin County, MN\"\t27053\n\"Wright County, MN\"\t27171\t\"McLeod County, MN\"\t27085\n\"Wright County, MN\"\t27171\t\"Meeker County, MN\"\t27093\n\"Wright County, MN\"\t27171\t\"Sherburne County, MN\"\t27141\n\"Wright County, MN\"\t27171\t\"Stearns County, MN\"\t27145\n\"Wright County, MN\"\t27171\t\"Wright County, MN\"\t27171\n\"Yellow Medicine County, MN\"\t27173\t\"Chippewa County, MN\"\t27023\n\"Yellow Medicine County, MN\"\t27173\t\"Lac qui Parle County, MN\"\t27073\n\"Yellow Medicine County, MN\"\t27173\t\"Lincoln County, MN\"\t27081\n\"Yellow Medicine County
